vi "main.vi"() -> ()   [LabVIEW 2018]
panel:
  out "PIP_GEN_id-0_2.0":string
  in  "XML File Path":path
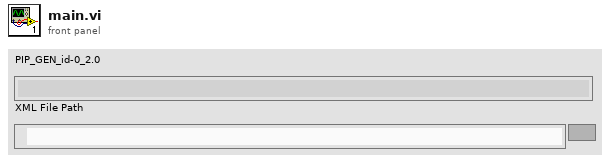
[diagram p1: front panel]
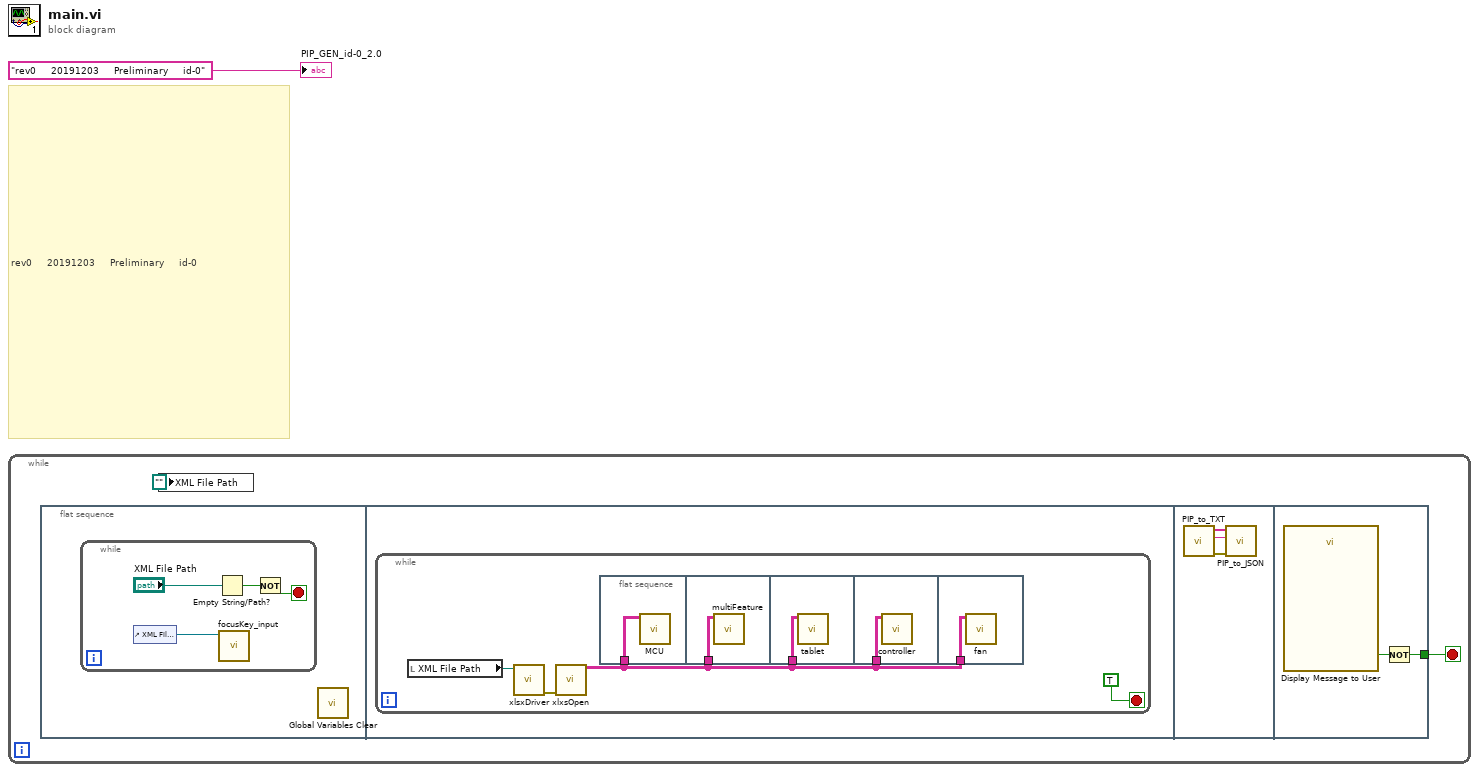
[diagram p0: block diagram]
diagram:
  # "rev0     20191203     Preliminary     id-0"
  n1 = while {
    stop <- w3 stop-if-true
    n2 = flat-sequence {
      tunnel: [w20] -> w3
      frame #0 {
        n3 = while {
          stop <- w4 stop-if-true
          n4 = control-ref of="XML File Path"() -> (w7:refnum<vi>)
          n5 = Empty String/Path?(string/path="XML File Path") -> (empty?=w5:bool)
          n6 = call "focusKey_input.vi"("reference"=w7) -> ()  [unwired: 10 in, 1 out]
          n7 = Not(x=w5) -> (.not. x?=w4:bool)
        }
        n8 = call "Global Variables Clear.vi"() -> ()  [unwired: 12 in]
      }
      frame #1 {
        n9 = while {
          stop <- TRUE stop-if-true
          n10 = local read "XML File Path"() -> (w9:path)
          n11 = call "xlsxDriver.vi"("XML File Path"=w9) -> ("error out"=w10:errorcluster)  [unwired: 10 in]
          n12 = call "xlxsOpen.vi"("error in (no error)"=w10) -> ("Shared_strings"=w8:string[][])  [unwired: 10 in, 4 out]
          n13 = flat-sequence {
            tunnel: w8 -> [w12]
            tunnel: w8 -> [w13]
            tunnel: w8 -> [w14]
            tunnel: w8 -> [w15]
            tunnel: w8 -> [w16]
            frame #0 {
              n14 = call "MCU.vi"("Shared_strings"=w12) -> ()  [unwired: 11 in]
            }
            frame #1 {
              n15 = call "multiFeature.vi"("Shared_strings"=w13) -> ()  [unwired: 11 in]
            }
            frame #2 {
              n16 = call "tablet.vi"("Shared_strings"=w14) -> ()  [unwired: 11 in]
            }
            frame #3 {
              n17 = call "controller.vi"("Shared_strings"=w15) -> ()  [unwired: 11 in]
            }
            frame #4 {
              n18 = call "fan.vi"("Shared_strings"=w16) -> ()  [unwired: 11 in]
            }
          }
        }
      }
      frame #2 {
        n19 = call "PIP_to_TXT.vi"() -> ("error out"=w17:errorcluster, "FileName"=w18:string, "PIP_to_JSN"=w19:string[])  [unwired: 9 in]
        n20 = call "PIP_to_JSON.vi"("error in (no error)"=w17, "FileName"=w18, "jsonGen"=w19) -> ()  [unwired: 8 in, 1 out]
      }
      frame #3 {
        n21 = call "Display Message to User"() -> ("YES"=w21:bool)  [unwired: 10 in, 1 out]
        n22 = Not(x=w21) -> (.not. x?=w20:bool)
      }
    }
    n23 = local write "XML File Path"(path "") -> ()
  }
  "PIP_GEN_id-0_2.0" <- "rev0     20191203     Preliminary     id-0"
